vi "New BS120x XNET Device.vi"(8 "error in (no error)":errorcluster, 9 "Box IDs":u8[](array[numeric]), 10 "CAN Interface":refnum<k21>, 11 "Unit Type":T1) -> (0 "error out":errorcluster, 3 "BS120x out":refnum<class "BS120x.lvclass">)   [LabVIEW 2021, in "BS120x Driver.lvlib"]
uses:
  BS120x Driver.lvlib
  TypeDefs/UnitType.ctl
  BS120x.lvclass
  CAN/XNET_BS120x.lvclass
  P:/_BLOOMY/7100-00109 SW BS1201 LV Driver/source/BS120x.lvclass
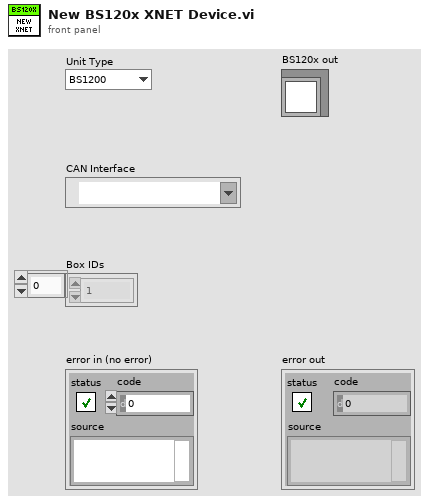
[diagram p1: front panel]
types:
  T1 = typedef "BS120x Driver.lvlib/BS120x.lvclass/UnitType.ctl" = enum16{"BS1200", "BS1201"}
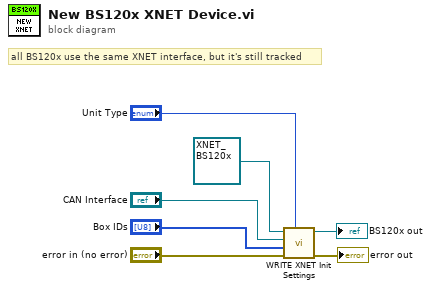
[diagram p0: block diagram]
diagram:
  # "all BS120x use the same XNET interface, but it's still tracked"
  n1 = call-dynamic "WRITE XNET Init Settings.vi"("Unit Type"="Unit Type", "error in (no error)"="error in (no error)", "Box IDs"="Box IDs", "CAN Interface"="CAN Interface", "XNET_BS120x in"=refnum<class "XNET_BS120x.lvclass"> refnum ("BS120x Driver.lvlib:XNET_BS120x.lvclass")) -> ("error out"=→"error out":errorcluster, "XNET_BS120x out"=→"BS120x out":refnum<class "XNET_BS120x.lvclass">)  [unwired: 5 in]
